vi "To table array.vi"(1 "Days":bool[][](array[boolean]), 2 "Costs":dbl[][](array[numeric]), 3 "Names":string[](array[string])) -> (0 "Table Array":string[][](array[string]))   [LabVIEW 2015]
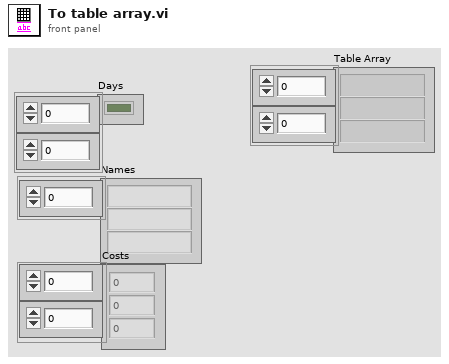
[diagram p1: front panel]
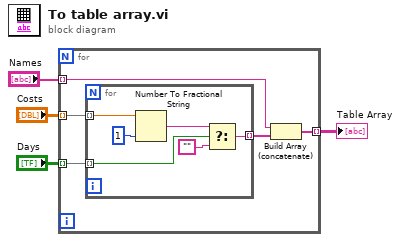
[diagram p0: block diagram]
diagram:
  n1 = for {
    tunnel: "Costs" -> [w6] mode=indexing
    tunnel: "Days" -> [w9] mode=indexing
    tunnel: [w8] -> w1 mode=indexing
    tunnel: "Names" -> [w7] mode=indexing
    n2 = for {
      tunnel: w9 -> [w15] mode=indexing
      tunnel: w6 -> [w14] mode=indexing
      tunnel: [w11] -> w5 mode=indexing
      n3 = Number To Fractional String(number=w14, precision (6)=i16 1) -> (F-format string=w12:string)  [unwired: 2 in]
      n4 = Select(t=w12, s=w15, f="") -> (s? t:f=w11:string)
    }
    n5 = Build Array (concatenate)(w7, w5) -> (w8:string[])
  }
  "Table Array" <- w1
